vi "Write Signal Generator.lvclass.vi"(10 "Signal Generator.lvclass":refnum<class "Signal Generator.lvclass">, 11 "RF Power in":refnum<class "RF Power.lvclass">) -> (3 "RF Power out":refnum<class "RF Power.lvclass">)   [LabVIEW 2020, in "RF Power.lvclass"]
uses:
  RF Power.lvclass
  Instruments/Signal Generator/Signal Generator.lvclass
  RF Power.lvclass/RF Power.ctl
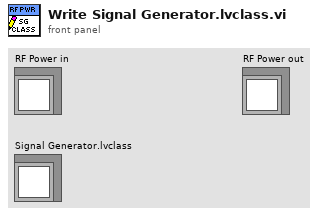
[diagram p1: front panel]
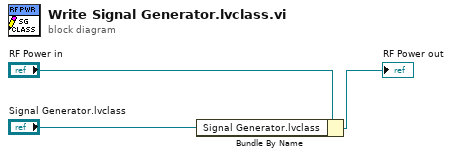
[diagram p0: block diagram]
diagram:
  n1 = Bundle By Name(cluster="RF Power in", "Signal Generator.lvclass"="Signal Generator.lvclass") -> (→"RF Power out":refnum<class "RF Power.lvclass">)
